vi "PROVA ESPORTA REPORT.vi"() -> ()   [LabVIEW 2019]
uses:
  <vilib>/addons/_office/excel.llb/Excel Easy Table (str).vi
  <vilib>/Utility/NIReport.llb/NI_report.lvclass
  <vilib>/Utility/NIReport.llb/Excel/NI_Excel.lvclass
  <vilib>/addons/_office/NI_ReportGenerationToolkit.lvlib
panel:
  out "error out 5":errorcluster
  out "error out 4":errorcluster
  out "error out 3":errorcluster
  out "error out 2":errorcluster
  out "error out":errorcluster
  in  "PDF":bool
  in  "XLS":bool
  in  "text data":string[][](array[string])=[["S", ""], ["", "S"]]
  in  "worksheet index (0)":i32
  in  "template (empty)":path
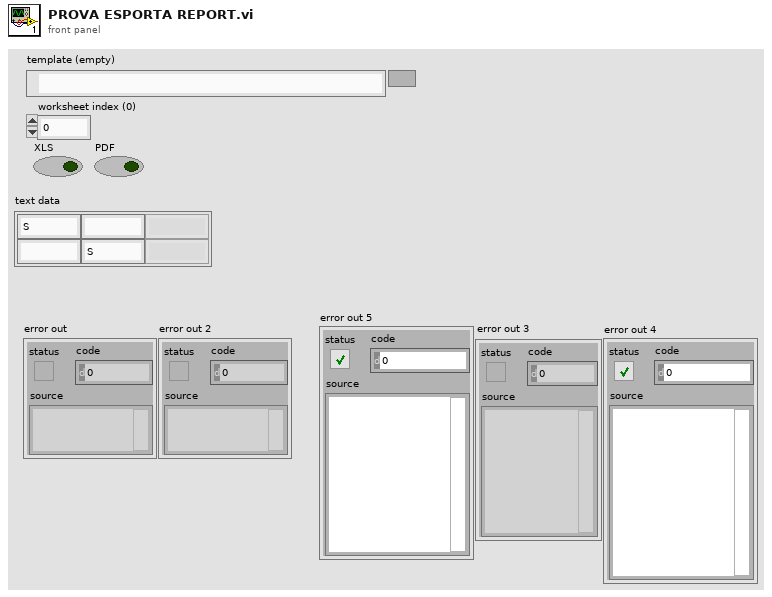
[diagram p1: front panel]
types:
  T1 = enum16{"maximized", "minimized", "normal", "no change"}
  T2 = enum16{"Standard Report", "HTML", "Word", "Excel"}
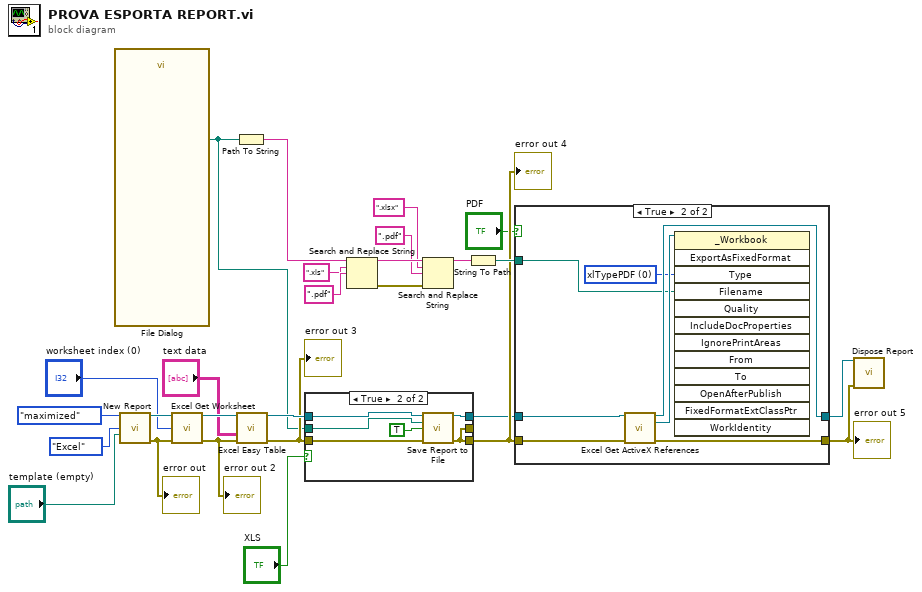
[diagram p0: block diagram]
diagram:
  n1 = call "File Dialog"() -> ("selected path"=w6:path)  [unwired: 7 in, 8 out]
  n2 = call <vilib>:"New Report.vi"("window state (normal)"=T1."maximized", "report type"=T2."Excel", "template (empty)"="template (empty)") -> ("report out"=w21:refnum<class "NI_report.lvclass">, "error out"=w22:errorcluster)  [unwired: 11 in]
  "error out" <- w22
  n3 = call <vilib>:"Excel Get Worksheet.vi"("report in"=w21, "worksheet index (0)"="worksheet index (0)", "error in (no error)"=w22) -> ("report out"=w20:refnum<class "NI_report.lvclass">, "error out"=w19:errorcluster)  [unwired: 11 in]
  "error out 2" <- w19
  n4 = Path To String(path=w6) -> (string=w7:string)
  n5 = call-poly <vilib>:"Excel Easy Table.vi"("report in"=w20, "text data"="text data", "error in (no error)"=w19) -> ("report out"=w18:refnum<class "NI_report.lvclass">, "error out"=w17:errorcluster)  [unwired: 8 in, 3 out]
  "error out 3" <- w17
  n6 = case shown="True" "XLS" {
    tunnel: w18 -> [w29 w34]
    tunnel: w17 -> [w28 w33]
    tunnel: [w29 w32] -> w3
    tunnel: [w28 w31] -> _
    tunnel: [w28 w31] -> w4
    tunnel: w6 -> [_ w30]
    frame False {
    }
    frame True {
      n7 = call-dynamic "Save Report to File.vi"("report in"=w34, "report file path"=w30, "prompt to replace? (F)"=TRUE, "error in (no error)"=w33) -> ("report out"=w32:refnum<class "NI_report.lvclass">, "error out"=w31:errorcluster)  [unwired: 10 in]
    }
  }
  "error out 4" <- w4
  n8 = Search and Replace String(input string=w7, search string=".xls", replace string=".pdf" ("replace string (\"\")")) -> (result string=w12:string, error out=w13:errorcluster)  [unwired: 5 in, 2 out]
  n9 = Search and Replace String(input string=w12, search string=".xlsx", replace string=".pdf" ("replace string (\"\")"), error in=w13) -> (result string=w14:string)  [unwired: 4 in, 3 out]
  n10 = String To Path(string=w14) -> (path=w5:path)
  n11 = case shown="True" "PDF" {
    tunnel: [w36 w42] -> w24
    tunnel: [w37 w43] -> w23
    tunnel: w5 -> [_ w40]
    tunnel: w4 -> [w36 w39]
    tunnel: w3 -> [w37 w38]
    frame False {
    }
    frame True {
      w41 = 0 items=["xlTypePDF", "xlTypeXPS"] ("Type")
      n12 = call <vilib>:"Excel Get ActiveX References.vi"("report in"=w38, "error in (no error)"=w39) -> ("report out"=w43:refnum<class "NI_report.lvclass">, "Excel._Workbook"=w44:refnum<k7>, "error out"=w42:errorcluster)  [unwired: 7 in, 4 out]
      n13 = invoke class="_Workbook" method="ExportAsFixedFormat"(reference=w44, "Type"=w41, "Filename"=w40) -> ()  [unwired: 10 in, 13 out]
    }
  }
  "error out 5" <- w24
  n14 = call-dynamic "Dispose Report.vi"("report in"=w23, "error in (no error)"=w24) -> ()  [unwired: 13 in, 1 out]
